vi "CheckRMXVersion.vi"(8 "error in (no error)":errorcluster, 11 "VISA resource name":refnum<visa-resource-name>) -> (0 "error out":errorcluster, 1 "Instrument Driver Revision":string, 2 "Instrument Firmware Revision":string, 3 "VISA resource name out":refnum<visa-resource-name>, 4 "RMXInformation":string)   [LabVIEW 2023]
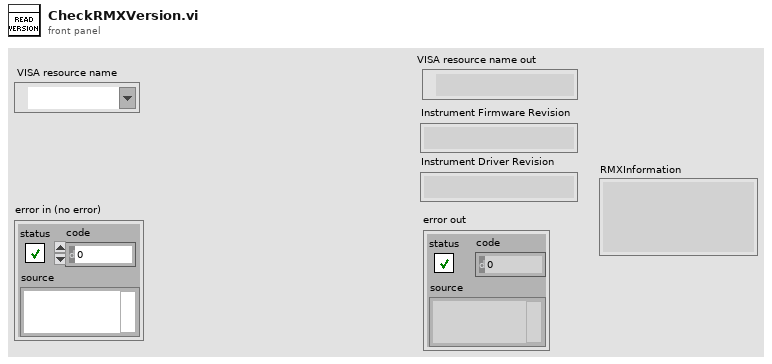
[diagram p1: front panel]
types:
  T1 = enum32{"invalid app kind", "Development System", "Run Time System", "Student Edition", "Embedded LabVIEW", "Evaluation", "Custom"}
  T2 = cluster{"Major":u16, "Minor":u16, "Fix":u16, "Build":u16}
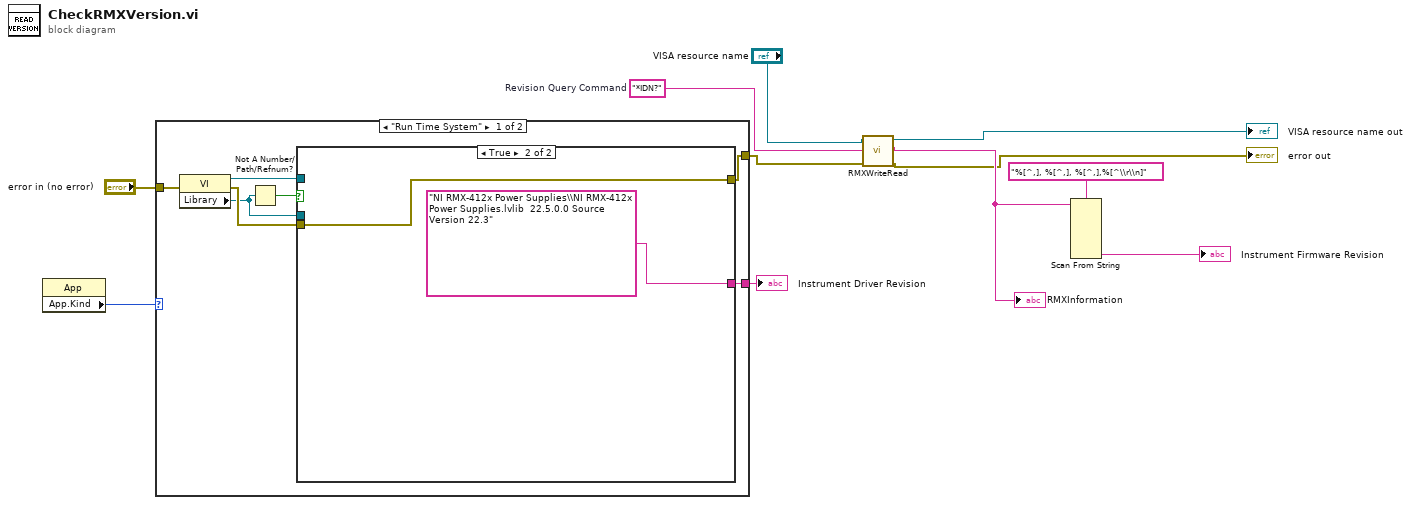
[diagram p0: block diagram]
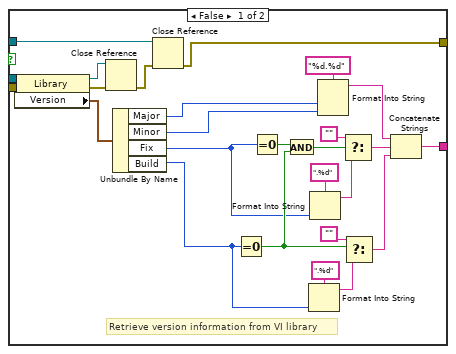
[diagram p2: hidden frame]
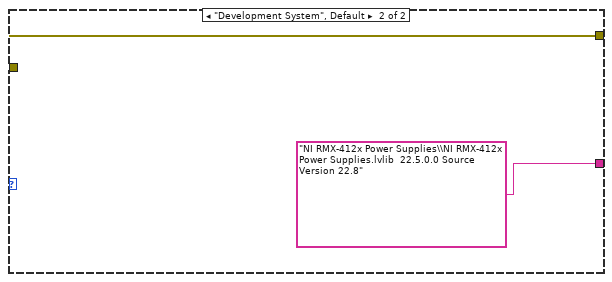
[diagram p3: hidden frame]
diagram:
  w5 = "*IDN?"  # Revision Query Command
  n1 = property class="App"() -> ("App.Kind"=w3:T1)  [unwired: 2 in, 2 out]
  n2 = case shown="\"Run Time System\"" w3 {
    tunnel: [w14 "NI RMX-412x Power Supplies\\NI RMX-412x Power Supplies.lvlib  22.5.0.0 Source Version 22.8"] -> w9
    tunnel: "error in (no error)" -> [w13 w48]
    tunnel: [w12 w48] -> w4
    frame "Run Time System" {
      n3 = property class="VI"(error in=w13) -> (reference out=w18:refnum<vi>, error out=w17:errorcluster, "Library"=w16:refnum<vi>)  [unwired: 1 in]
      n4 = Not A Number/Path/Refnum?(number/path/refnum=w16) -> (NaN/Path/Refnum?=w15:bool)
      n5 = case shown="True" w15 {
        tunnel: w18 -> [w41 _]
        tunnel: w17 -> [w30 w46]
        tunnel: [w26 w46] -> w12
        tunnel: [w25 "NI RMX-412x Power Supplies\\NI RMX-412x Power Supplies.lvlib  22.5.0.0 Source Version 22.3"] -> w14
        tunnel: w16 -> [w24 _]
        frame False {
          # "Retrieve version information from VI library"
          n6 = property class="Library"(reference=w24, error in=w30) -> (reference out=w43:refnum<vi>, error out=w44:errorcluster, "Version"=w19:T2)
          n7 = Close Reference(reference=w43, error in (no error)=w44) -> (error out=w42:errorcluster)
          n8 = Unbundle By Name(w19) -> ("Major"=w23:u16, "Minor"=w22:u16, "Fix"=w21:u16, "Build"=w20:u16)
          n9 = Close Reference(reference=w41, error in (no error)=w42) -> (error out=w26:errorcluster)
          n10 = Equal To 0?(x=w20) -> (x = 0?=w28:bool)
          n11 = Equal To 0?(x=w21) -> (x = 0?=w29:bool)
          n12 = And(x=w29, y=w28) -> (x .and. y?=w27:bool)
          n13 = Format Into String(format string=".%d", w20) -> (resulting string=w34:string)  [unwired: 2 in, 1 out]
          n14 = Format Into String(format string=".%d", w21) -> (resulting string=w38:string)  [unwired: 2 in, 1 out]
          n15 = Format Into String(format string="%d.%d", w23, w22) -> (resulting string=w36:string)  [unwired: 2 in, 1 out]
          n16 = Select(t="", s=w27, f=w38) -> (s? t:f=w35:string)
          n17 = Select(t="", s=w28, f=w34) -> (s? t:f=w31:string)
          n18 = Concatenate Strings(w36, w35, w31) -> (w25:string)
        }
        frame True {
        }
      }
    }
    frame "Development System", Default {
    }
  }
  "Instrument Driver Revision" <- w9
  n19 = call "RMXWriteRead.vi"("error in (no error)"=w4, "Write Command/Query"=w5, "VISA resource name"="VISA resource name") -> ("error out"=→"error out":errorcluster, "Response"=w6:string, "VISA resource name out"=→"VISA resource name out":refnum<visa-resource-name>)  [unwired: 6 in]
  "RMXInformation" <- w6
  n20 = Scan From String(format string="%[^,], %[^,], %[^,],%[^\\r\\n]", input string=w6) -> (output 4=→"Instrument Firmware Revision":string)  [unwired: 9 in, 3 out]
